vi "军蚁-引导算角度2.vi"(0 "Image in":T9(plugin-control), 2 "Options":T8={"Search Direction"=3, "Edge Options"={"Edge Polarity"=0, "Kernel Size"=3, "Width"=3, "Minimum Edge Strength"=50.0, "Interpolation Type"=enum."Bilinear Fixed", "Data Processing Method"=enum."Average"}, "Show Search Area"=TRUE, "Show Search Lines"=TRUE, "Show Edges Found"=TRUE, "Show Result"=TRUE, "Search Area Color"=65280, "Search Lines Color"=255, "Edge Locations Color"=16776960, "Result Color"=16711680, "Overlay Group Name"=""} {"Search Direction" items=["Left to Right", "Right to Left", "Top to Bottom", "Bottom to Top"]; "Edge Options"."Edge Polarity" items=["All Edges", "Rising Edges", "Falling Edges"]; "Edge Options"."Minimum Edge Strength" format="%.2f"; "Edge Options"."Width" step=2; "Edge Options"."Kernel Size" step=2}, 3 "Fit Options":T4={"Number of Lines"=1, "Type"=enum."First Edge Rake", "Min. Score"=10.0, "Max. Score"=1000.0, "Orientation"=0.0, "Angle Range"=45.0, "Angle Tolerance"=1.0, "Step Size"=64, "Min. SNR (db)"=0.0, "Min. Points (%)"=25.0, "Hough Iterations"=5} {"Min. Points (%)" min=0.0 max=100.0; "Min. SNR (db)" min=0.0; "Max. Score" min=0.0 max=1024.0; "Min. Score" min=0.0 max=1024.0 step=1.0}, 4 "ROI Descriptor":T3={"Global Rectangle"=[915, 72, 1558, 856], "Contours"=[{"ID"=enum."External", "Type"=12, "Coordinates"=[915, 72, 1558, 856, 0]}]} {"Contours"."Type" items=["No Selection", "Point", "Line", "Rectangle", "Oval", "Polygon", "Freehand Region", "Annulus", "Unused2", "Unused3", "Broken Line", "Freehand Line", "Rotated Rectangle"]}, 7 "error in":errorcluster) -> (20 "Image Out":T9(plugin-control), 21 "Angle (Pixel)":dbl, 27 "error out":errorcluster)   [LabVIEW 2017]
uses:
  <vilib>/vision/Measure.llb/Edge Options.ctl
  <vilib>/vision/Measure.llb/Edge Polarity.ctl
  <vilib>/vision/Measure.llb/Straight Edge Options.ctl
  <vilib>/vision/Measure.llb/Straight Edge Process.ctl
  Global System.vi
  <vilib>/vision/NI_Vision_Development_Module.lvlib
panel:
  in  "Reference System":T1={"Origin"={"X"=1030.3278, "Y"=941.8893}, "Angle (deg)"=354.93622, "Axis Reference"=0} {"Axis Reference" items=["Direct", "Indirect"]}
  out "输出簇":T1
  out "Cluster":T2
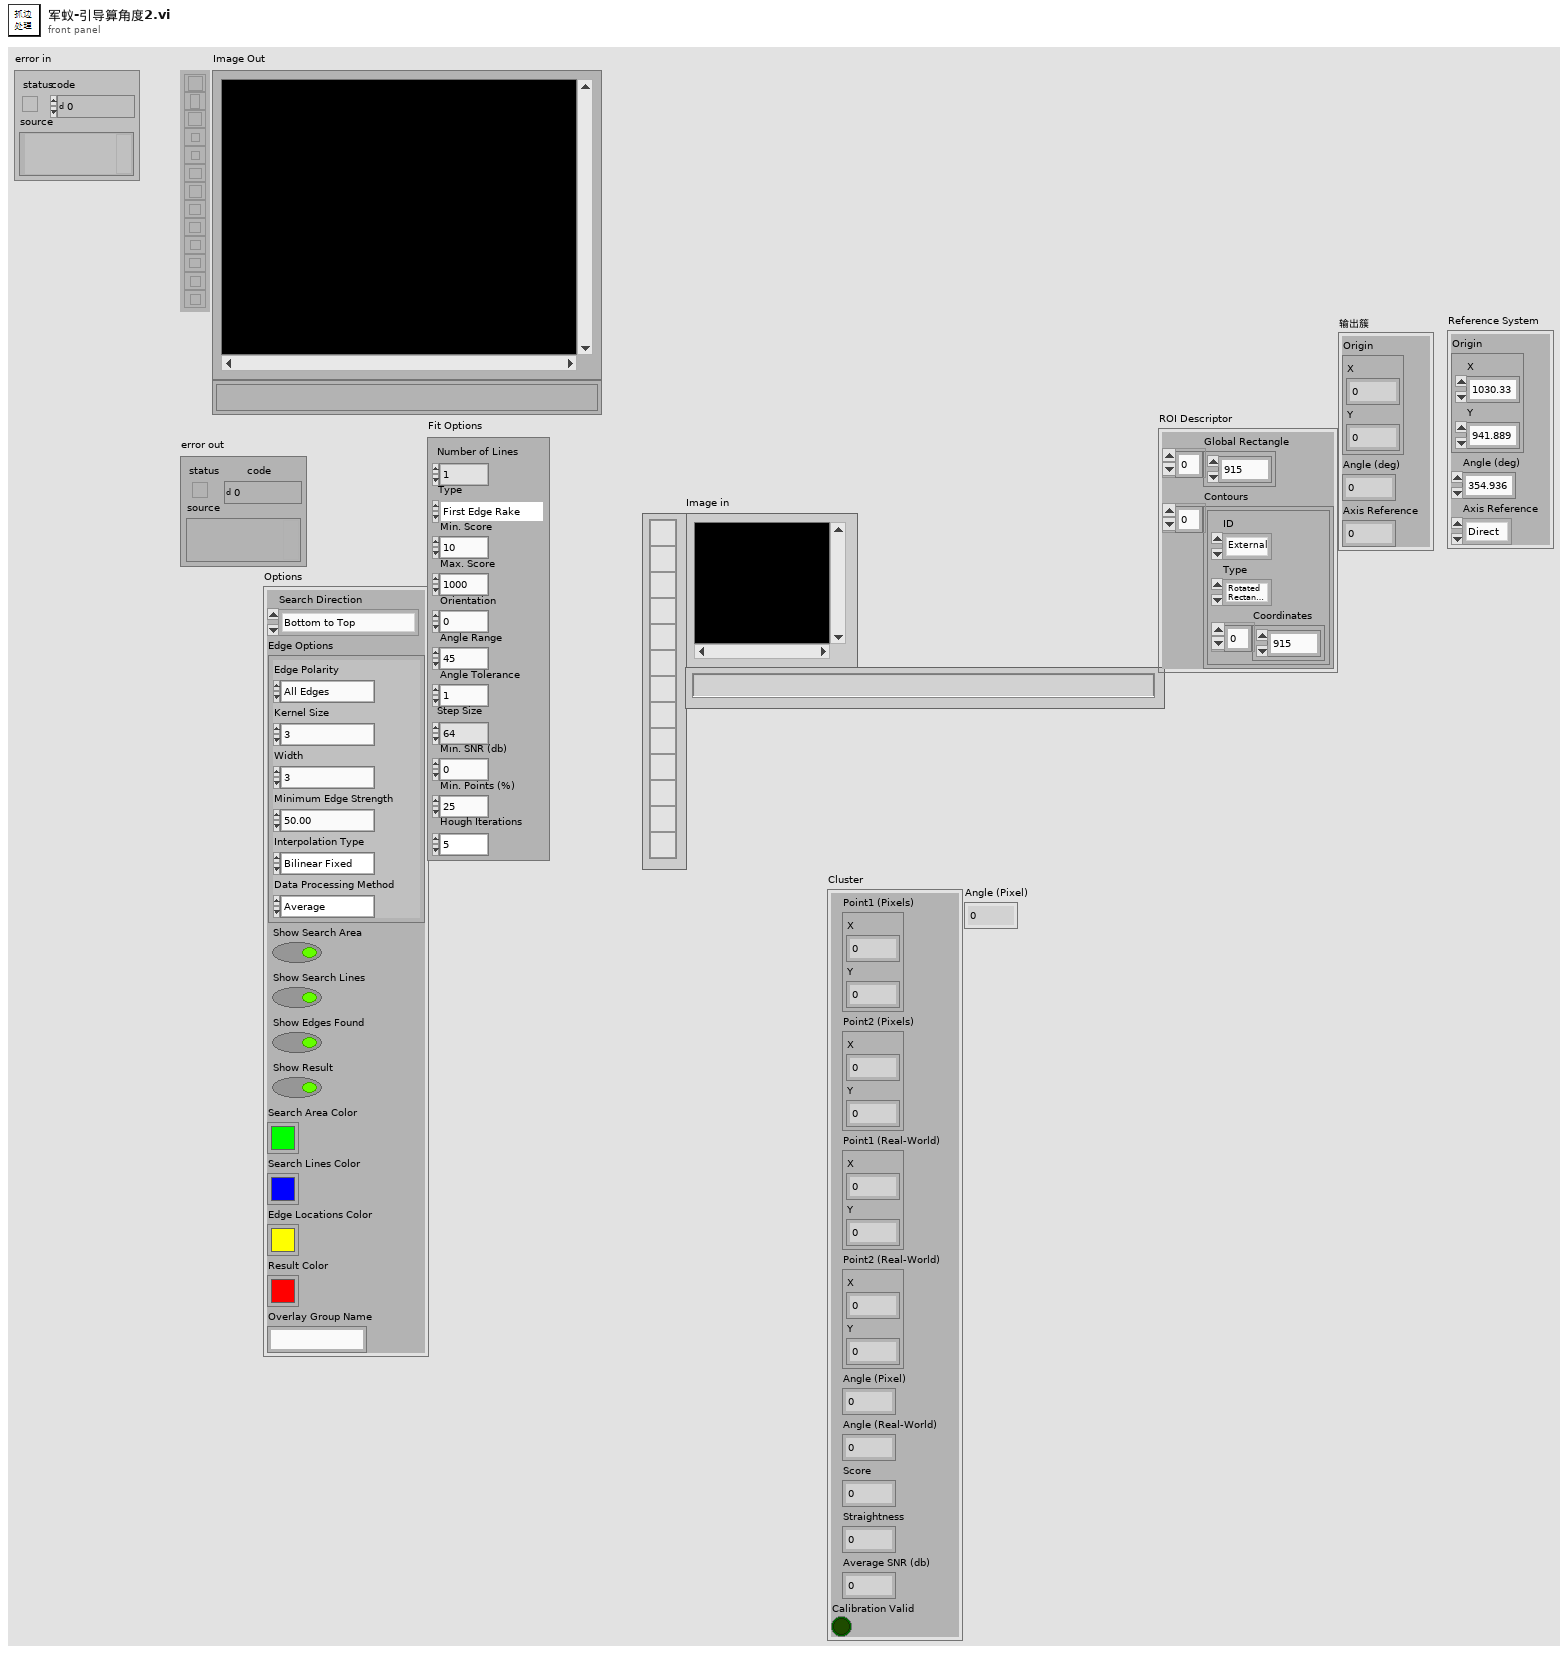
[diagram p1: front panel]
types:
  T1 = cluster{"Origin":cluster{"X":sgl, "Y":sgl}, "Angle (deg)":sgl, "Axis Reference":u32}
  T2 = cluster{"Point1 (Pixels)":cluster{"X":sgl, "Y":sgl}, "Point2 (Pixels)":cluster{"X":sgl, "Y":sgl}, "Point1 (Real-World)":cluster{"X":sgl, "Y":sgl}, "Point2 (Real-World)":cluster{"X":sgl, "Y":sgl}, "Angle (Pixel)":dbl, "Angle (Real-World)":dbl, "Score":dbl, "Straightness":dbl, "Average SNR (db)":dbl, "Calibration Valid":bool}
  T3 = cluster{"Global Rectangle":i32[], "Contours":cluster{"ID":enum32{"External", "Internal"}, "Type":u32, "Coordinates":i32[]}[]}
  T4 = typedef "Straight Edge Options.ctl" = cluster{"Number of Lines":i32, "Type":T5, "Min. Score":dbl, "Max. Score":dbl, "Orientation":dbl, "Angle Range":dbl, "Angle Tolerance":dbl, "Step Size":u32, "Min. SNR (db)":dbl, "Min. Points (%)":dbl, "Hough Iterations":i32}
  T5 = typedef "Straight Edge Process.ctl" = enum32{"First Edge Rake", "Best Edge Rake", "Hough Edge Rake", "First Edge Projection", "Best Edge Projection"}
  T6 = typedef "Edge Options.ctl" = cluster{"Edge Polarity":T7, "Kernel Size":u32, "Width":u32, "Minimum Edge Strength":sgl, "Interpolation Type":enum32{"Zero Order", "Bilinear", "Quadratic", "Cubic", "Bilinear Fixed"}, "Data Processing Method":enum32{"Average", "Median"}}
  T7 = typedef "Edge Polarity.ctl" = u32
  T8 = cluster{"Search Direction":u32, "Edge Options":T6, "Show Search Area":bool, "Show Search Lines":bool, "Show Edges Found":bool, "Show Result":bool, "Search Area Color":u32, "Search Lines Color":u32, "Edge Locations Color":u32, "Result Color":u32, "Overlay Group Name":string}
  T9 = typedef "IMAQ Image.ctl" = refnum<image>
  T10 = cluster{"Desired Font (Application)":enum16{"User-specified Font", "Application Font", "System Font", "Dialog Font"}, "[User-specified Font]":cluster{"Font Name":string, "Size":i16, "Strikeout?":bool, "Italic?":bool, "Underline?":bool, "Outline?":bool, "Shadow?":bool, "Bold?":bool, "Rotation Angle":dbl}, "Horizontal Alignment":i16, "Vertical Alignment":i16}
  T11 = enum16{"Reset", "Update Coordinate System", "Get Coordinate System"}
  T12 = enum16{"Horizontal Motion", "Vertical Motion", "Horizontal and Vertical Motion", "Horizontal, Vertical and Angular Motion"}
  T13 = typedef "IMAQ Coordinate System" = cluster{"Reference System":cluster{"Origin":cluster{"X":sgl, "Y":sgl}, "Angle (deg)":sgl, "Axis Reference":u32}, "Measurement System":cluster{"Origin":cluster{"X":sgl, "Y":sgl}, "Angle (deg)":sgl, "Axis Reference":u32}}
  T14 = typedef "ROI Descriptor" = cluster{"Global Rectangle":i32[], "Contours":cluster{"ID":enum32{"External", "Internal"}, "Type":u32, "Coordinates":i32[]}[]}
  T15 = cluster{"Point1 (Pixels)":cluster{"X":sgl, "Y":sgl}, "Point2 (Pixels)":cluster{"X":sgl, "Y":sgl}, "Point1 (Real-World)":cluster{"X":sgl, "Y":sgl}, "Point2 (Real-World)":cluster{"X":sgl, "Y":sgl}, "Angle (Pixel)":dbl, "Angle (Real-World)":dbl, "Score":dbl, "Straightness":dbl, "Average SNR (db)":dbl, "Calibration Valid":bool}[]
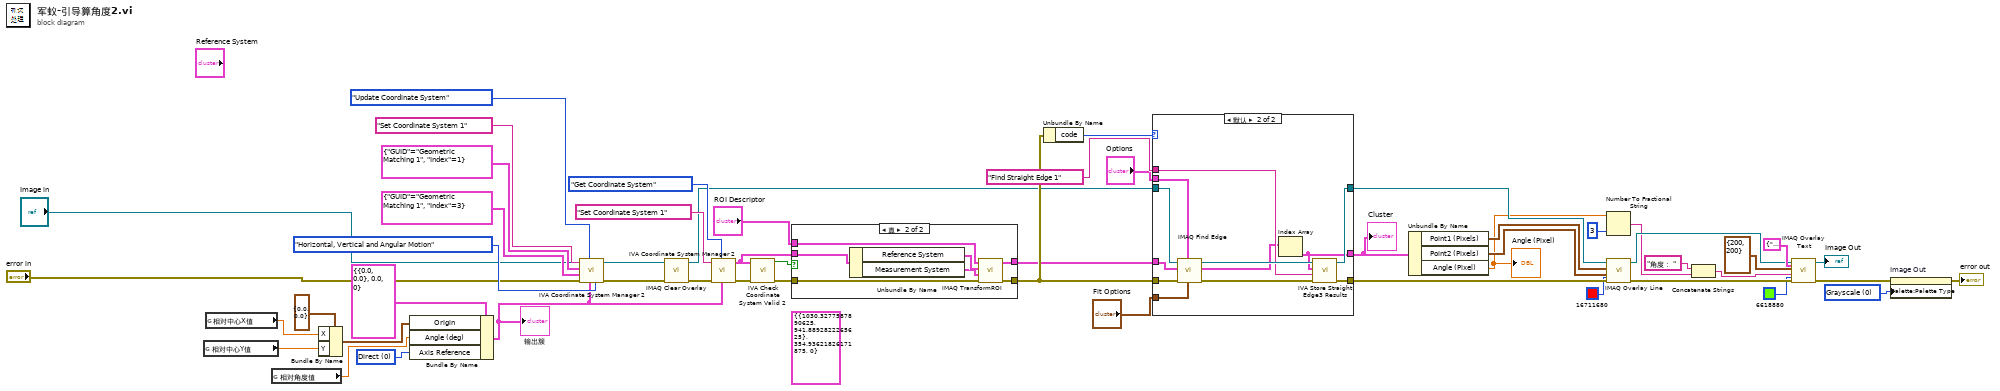
[diagram p0: block diagram]
diagram:
  (unwired) T1 {"Origin"={"X"=1030.3278, "Y"=941.8893}, "Angle (deg)"=354.93622, "Axis Reference"=0} ("Reference System")
  w25 = u32 0 items=["Direct", "Indirect"] ("Axis Reference")
  w32 = u32 0 items=["Grayscale", "Binary", "Gradient", "Rainbow", "Temperature", "User Defined", "Binary 16 Bit", "Gradient 16 Bit", "Rainbow 16 Bit", "Temperature 16 Bit", "User Defined 16 Bit"] ("Palette Type")
  n1 = global read "Global System.vi" "相对中心Y值"() -> (w28:dbl)
  n2 = global read "Global System.vi" "相对中心X值"() -> (w29:dbl)
  n3 = global read "Global System.vi" "相对角度值"() -> (w26:dbl)
  n4 = Bundle By Name(cluster=cluster{"X":sgl, "Y":sgl} {"X"=0.0, "Y"=0.0} ("Origin"), "X"=w29, "Y"=w28) -> (w27:cluster{"X":sgl, "Y":sgl})
  n5 = Bundle By Name(cluster=T1 {"Origin"={"X"=0.0, "Y"=0.0}, "Angle (deg)"=0.0, "Axis Reference"=0} ("Reference System"), "Origin"=w27, "Angle (deg)"=w26, "Axis Reference"=w25) -> (w23:T1)
  "输出簇" <- w23
  n6 = call <vilib>:"IVA Coordinate System Manager 2.vi"("Mode"=T12."Horizontal, Vertical and Angular Motion", "Reference System"=w23, "Function"=T11."Update Coordinate System", "error in (no error)"="error in", "Angle ID"=cluster{"GUID":string, "Index":i32} {"GUID"="Geometric Matching 1", "Index"=3}, "Origin ID"=cluster{"GUID":string, "Index":i32} {"GUID"="Geometric Matching 1", "Index"=1}, "Coordinate System Name"="Set Coordinate System 1") -> ("error out"=w22:errorcluster)  [unwired: 4 out]
  n7 = call "IMAQ Clear Overlay"("error in (no error)"=w22, "Image"="Image in") -> ("error out"=w19:errorcluster, "Image Out"=w20:T9)  [unwired: 8 in]
  n8 = call <vilib>:"IVA Coordinate System Manager 2.vi"("Reference System"=w23, "Function"=T11."Get Coordinate System", "error in (no error)"=w19, "Coordinate System Name"="Set Coordinate System 1") -> ("error out"=w44:errorcluster, "Coordinate System Out"=w41:T13)  [unwired: 3 in, 3 out]
  n9 = call <vilib>:"IVA Check Coordinate System Valid 2.vi"("error in (no error)"=w44, "Coordinate System"=w41) -> ("error out"=w39:errorcluster, "Valid?"=w40:bool)  [unwired: 8 out]
  n10 = case "条件结构" shown="真" w40 {
    tunnel: "ROI Descriptor" -> [w53 w60]
    tunnel: [w53 w57] -> w38
    tunnel: [w52 w56] -> w42
    tunnel: w41 -> [_ w55]
    tunnel: w39 -> [w52 w54]
    frame False {
    }
    frame True {
      n11 = Unbundle By Name(w55) -> ("Reference System"=w59:T1, "Measurement System"=w58:T1)
      n12 = call "IMAQ TransformROI"("error in (no error)"=w54, "New Reference"=w58, "Base Reference"=w59, "ROI Descriptor"=w60) -> ("error out"=w56:errorcluster, "ROI Descriptor out"=w57:T14)  [unwired: 6 out]
    }
  }
  n13 = Unbundle By Name(w42) -> ("code"=w36:i32)
  n14 = case "条件结构" shown="默认" w36 {
    tunnel: w20 -> [w61 w73]
    tunnel: w42 -> [_ w72]
    tunnel: w38 -> [_ w66]
    tunnel: [w61 w70] -> w17
    tunnel: [_ w68] -> w16
    tunnel: "Find Straight Edge 1" ("Step Name") -> [_ w67]
    tunnel: "Fit Options" -> [_ w65]
    tunnel: "Options" -> [_ w64]
    tunnel: [_ w62] -> w18
    frame -1074396199, -1074396198 {
      # "Discard Coordinate System Error"
    }
    frame Default {
      n15 = call "IMAQ Find Edge"("Line Fit Options"=w65, "Options"=w64, "error in (no error)"=w72, "ROI Descriptor"=w66, "Image"=w73) -> ("error out"=w69:errorcluster, "Straight Edges"=w63:T15, "Image Out"=w71:T9)  [unwired: 1 in, 3 out]
      n16 = Index Array(array=w63) -> (element=w62:T2)  [unwired: 1 in]
      n17 = call <vilib>:"IVA Store Straight Edge3 Results.vi"("error in (no error)"=w69, "Step Name"=w67, "Straight Edge"=w62, "Image in"=w71) -> ("error out"=w68:errorcluster, "Image dup"=w70:T9)  [unwired: 1 in, 5 out]
    }
  }
  "Cluster" <- w18
  n18 = Unbundle By Name(w18) -> ("Point1 (Pixels)"=w15:cluster{"X":sgl, "Y":sgl}, "Point2 (Pixels)"=w14:cluster{"X":sgl, "Y":sgl}, "Angle (Pixel)"=w6:dbl)
  "Angle (Pixel)" <- w6
  n19 = Number To Fractional String(number=w6, precision (6)=i16 3 ("精度(6)")) -> (F-format string=w3:string)  [unwired: 2 in]
  n20 = call "IMAQ Overlay Line"("Color"=u32 16711680, "error in (no error)"=w16, "End Point"=w14, "Start Point"=w15, "Image"=w17) -> ("error out"=w8:errorcluster, "Image Out"=w10:T9)  [unwired: 5 in]
  n21 = Concatenate Strings("角度： " ("字符串"), w3) -> (w2:string)
  n22 = call "IMAQ Overlay Text"("Text Color (black)"=u32 6618880, "Font, Size & Style"=T10 {"Desired Font (Application)"=enum."User-specified Font", "[User-specified Font]"={"Font Name"="", "Size"=100, "Strikeout?"=FALSE, "Italic?"=FALSE, "Underline?"=FALSE, "Outline?"=FALSE, "Shadow?"=FALSE, "Bold?"=TRUE, "Rotation Angle"=0.0}, "Horizontal Alignment"=0, "Vertical Alignment"=0}, "error in (no error)"=w8, "String"=w2, "Origin"=cluster{"X":i32, "Y":i32} {"X"=200, "Y"=200}, "Image"=w10) -> ("error out"=w7:errorcluster, "Image Out"=→"Image Out":T9)  [unwired: 4 in]
  n23 = property on="Image Out" class="ImageControl"(error in=w7, "Palette:Palette Type"=w32) -> (error out=→"error out":errorcluster)  [unwired: 1 in, 1 out]
